vi "Test - Is String Constant a State Constant.vi"() -> ()   [LabVIEW 2013, in "JKI State Machine API - Tests.lvlib"]
uses:
  tests/JKI State Machine API - Tests.lvlib
  <vilib>/Utility/traverseref.llb/TRef TravTarget.ctl
  <vilib>/Utility/traverseref.llb/VI Scripting - Traverse.lvlib
  JKI State Machine API.lvlib
  JKI SM/JKI SM.lvclass
panel:
  out "error out":errorcluster
  out "States":string[](array[string])
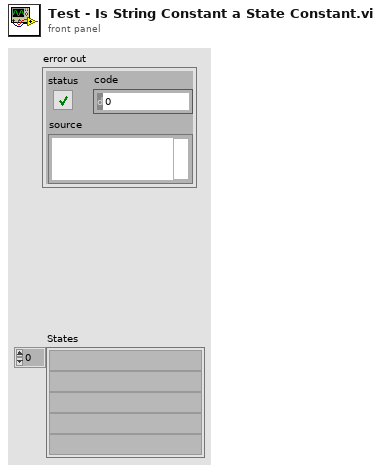
[diagram p1: front panel]
types:
  T1 = typedef "TRef TravTarget.ctl" = enum16{"FP", "BD", "Other"}
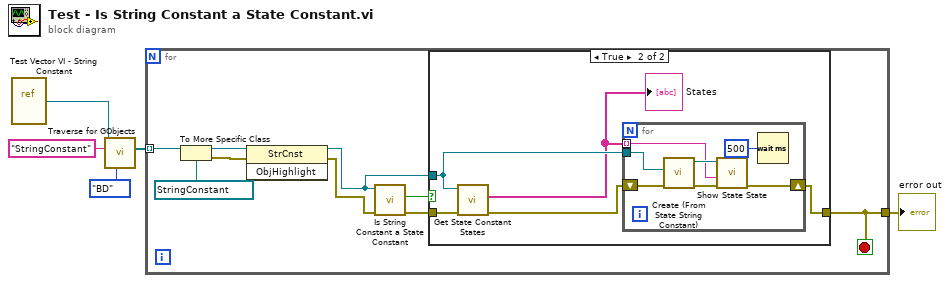
[diagram p0: block diagram]
diagram:
  n1 = vi-ref "Test Vector VI - String Constant.vi"() -> (w5:refnum<vi>)
  n2 = call <vilib>:"Traverse for GObjects.vi"("Traverse Target"=TRef_TravTarget."BD", "Class Name"="StringConstant", "VI Refnum"=w5) -> ("References"=w2:refnum<vi>[])  [unwired: 5 in, 3 out]
  n3 = for {
    tunnel: w2 -> [w13] mode=indexing
    tunnel: [w6] -> w1
    stop <- w6 stop-if-true
    n4 = To More Specific Class(target class=refnum<vi> refnum ("StrCnst Refnum"), reference=w13) -> (specific class reference=w10:refnum<vi>, error out=w8:errorcluster)  [unwired: 1 in]
    n5 = invoke class="StrCnst" method="ObjHighlight"(reference=w10, error in=w8) -> (reference out=w9:refnum<vi>, error out=w7:errorcluster)  [unwired: 1 in, 1 out]
    n6 = call "Is String Constant a State Constant.vi"("error in (no error)"=w7, "StrCnst Refnum"=w9) -> ("error out"=w11:errorcluster, "Is States Constant"=w12:bool)  [unwired: 7 in, 1 out]
    n7 = case shown="True" w12 {
      tunnel: w9 -> [_ w19]
      tunnel: w11 -> [w15 w20]
      tunnel: [w15 w16] -> w6
      frame False {
      }
      frame True {
        n8 = call "Get State Constant States.vi"("error in (no error)"=w20, "StrCnst Refnum"=w19) -> ("error out"=w18:errorcluster, "States"=w17:string[])  [unwired: 8 in]
        "States" <- w17
        n9 = for {
          shift-right: [w24] -> w16
          shift-left: w18 -> [w25]
          tunnel: w19 -> [w23]
          tunnel: w17 -> [w22] mode=indexing
          n10 = call "Create (From State String Constant).vi"("error in (no error)"=w25, "State String Constant"=w23) -> ("error out"=w26:errorcluster, "JKI SM out"=w27:refnum<class "JKI SM.lvclass">)  [unwired: 6 in, 2 out]
          n11 = call "Show State State.vi"("error in (no error)"=w26, "State Name"=w22, "JKI SM in"=w27) -> ("error out"=w24:errorcluster)  [unwired: 7 in, 1 out]
          n12 = Wait (ms)(milliseconds to wait=u32 500) -> ()  [unwired: 1 out]
        }
      }
    }
  }
  "error out" <- w1
